vi "DMA.Concatenate Block.vi"(10 "New Block":T1 {"size" format="%08x"; "pointer" format="%08x"}, 11 "DMA Blocks":T1[](array[typedef]) {"size" format="%08x"; "pointer" format="%08x"}) -> (1 "block index":i32, 3 "DMA Blocks out":T1[](array[typedef]) {"size" format="%08x"; "pointer" format="%08x"})   [LabVIEW 2016, in "GE 5565PIORC.lvclass"]
uses:
  GE 5565PIORC.lvclass
  Controls/DMA Block.ctl
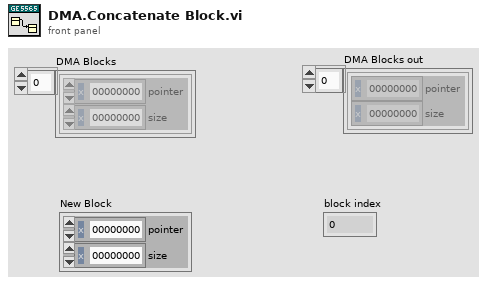
[diagram p1: front panel]
types:
  T1 = typedef "GE 5565PIORC.lvclass/DMA Block.ctl" = cluster{"pointer":u32, "size":u32}
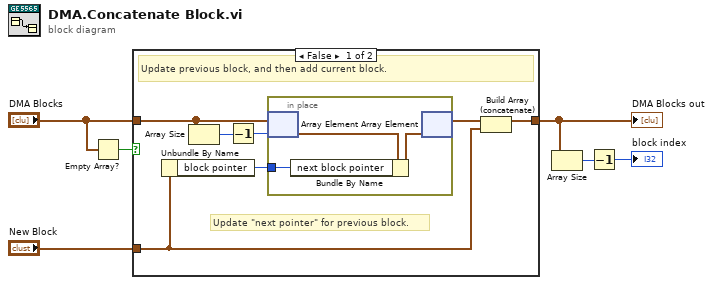
[diagram p0: block diagram]
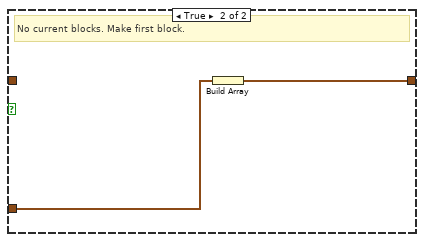
[diagram p2: hidden frame]
diagram:
  n1 = Empty Array?(array="DMA Blocks") -> (empty?=w5:bool)
  n2 = case shown="False" w5 {
    tunnel: "DMA Blocks" -> [w8 _]
    tunnel: "New Block" -> [w10 w17]
    tunnel: [w9 w18] -> w3
    frame False {
      # "Update \"next pointer\" for previous block."
      # "Update previous block, and then add current block."
      n3 = Unbundle By Name(w10) -> ("block pointer"=w12:u32)
      n4 = Array Size(array=w8) -> (size(s)=w7:i32)
      n5 = Decrement(x=w7) -> (x-1=w13:i32)
      n6 = in-place {
        in-place-border: w12 -> [w14]
        n7 = in-place-array #1(w8, w13) -> (w16:T1)
        n8 = Bundle By Name(cluster=w16, "next block pointer"=w14) -> (w15:T1)
        n9 = in-place-array #1(w15) -> (w11:T1[])  [unwired: 1 out]
      }
      n10 = Build Array (concatenate)(w11, w10) -> (w9:T1[])
    }
    frame True {
      # "No current blocks. Make first block."
      n11 = Build Array(w17) -> (w18:T1[])
    }
  }
  "DMA Blocks out" <- w3
  n12 = Array Size(array=w3) -> (size(s)=w2:i32)
  n13 = Decrement(x=w2) -> (x-1=→"block index":i32)
